vi "Module Init.vi"(8 "error in (no error)":errorcluster, 11 "System Status Module in":refnum<class "System Status Module.lvclass">) -> (0 "error out":errorcluster, 3 "System Status Module out":refnum<class "System Status Module.lvclass">)   [LabVIEW 2020, in "VolatusGUI.lvlib" / "System Status Module.lvclass"]
uses:
  System Status Module.lvclass
  C:/dev/lv20CE/relink/lv-volatus/Volatus/Module/Module.lvclass
  Volatus/Module/Module.lvclass/Module.ctl
  Volatus/MessageQ/MessageQ.lvclass/MessageQ.ctl
  Volatus/Module/Self Q.vi
  Volatus/MessageQ/Send.vi
  System Status Module.lvclass/System Status Module.ctl
  Volatus/Module/Module.lvclass
  C:/dev/lv20CE/relink/lv-volatus/VolatusGUI/System Status Module/System Status Module.lvclass
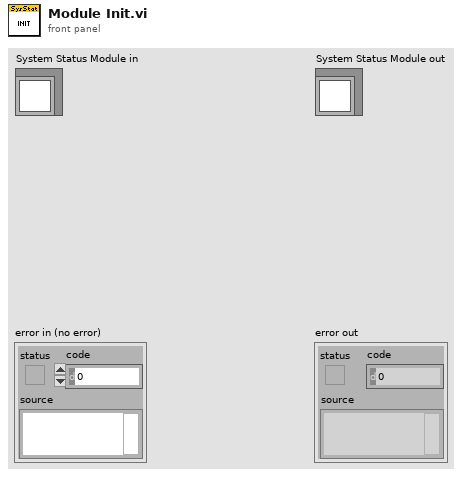
[diagram p1: front panel]
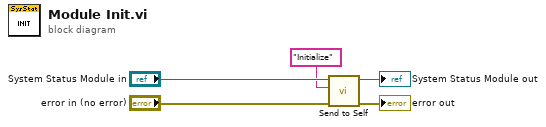
[diagram p0: block diagram]
diagram:
  n1 = call "Send to Self.vi"("error in (no error)"="error in (no error)", "Message ID"="Initialize", "Module in"="System Status Module in") -> ("error out"=→"error out":errorcluster, "Module out"=→"System Status Module out":refnum<class "System Status Module.lvclass">)  [unwired: 7 in]
